vi "LEP_RV_MemoryMap_Default.vi"(8 "error in (no error)":errorcluster, 11 "VI Path":path) -> (0 "error out":errorcluster, 3 "VI Config":T1)   [LabVIEW 2011]
doc: "Define default memory mapping for the Axiom CMD565 target."
uses:
  <vilib>/LabVIEW Targets/Embedded/Utilities/MemMap/EMB_Utility_MemMap_VI_Config.ctl
  <vilib>/LabVIEW Targets/Embedded/Utilities/MemMap/EMB_Utility_MemMap_VI_Type.ctl
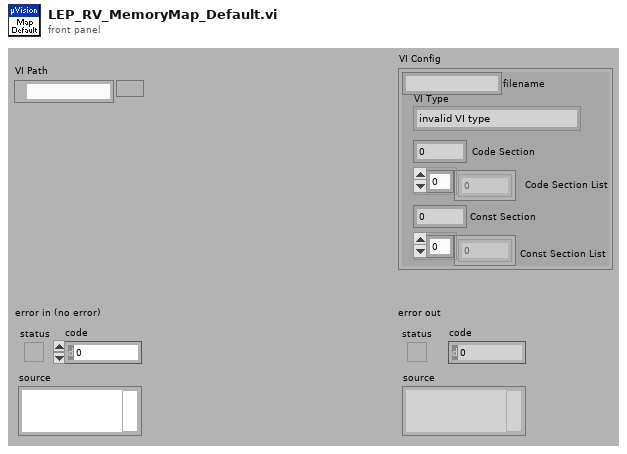
[diagram p1: front panel]
types:
  T1 = typedef "EMB_Utility_MemMap_VI_Config.ctl" = cluster{"filename":string, "Code Section":i32, "Code Section List":i32[], "Const Section":i32, "Const Section List":i32[], "VI Type":T2}
  T2 = typedef "EMB_Utility_MemMap_VI_Type.ctl" = enum32{"invalid VI type", "Standard VI", "Control VI", "Global VI", "Polymorphic VI", "Configuration VI", "SubSystem"}
  T3 = enum32{"invalid VI type", "Standard VI", "Control VI", "Global VI", "Polymorphic VI", "Configuration VI", "SubSystem", "Facade VI", "Method VI", "Statechart Diagram VI"}
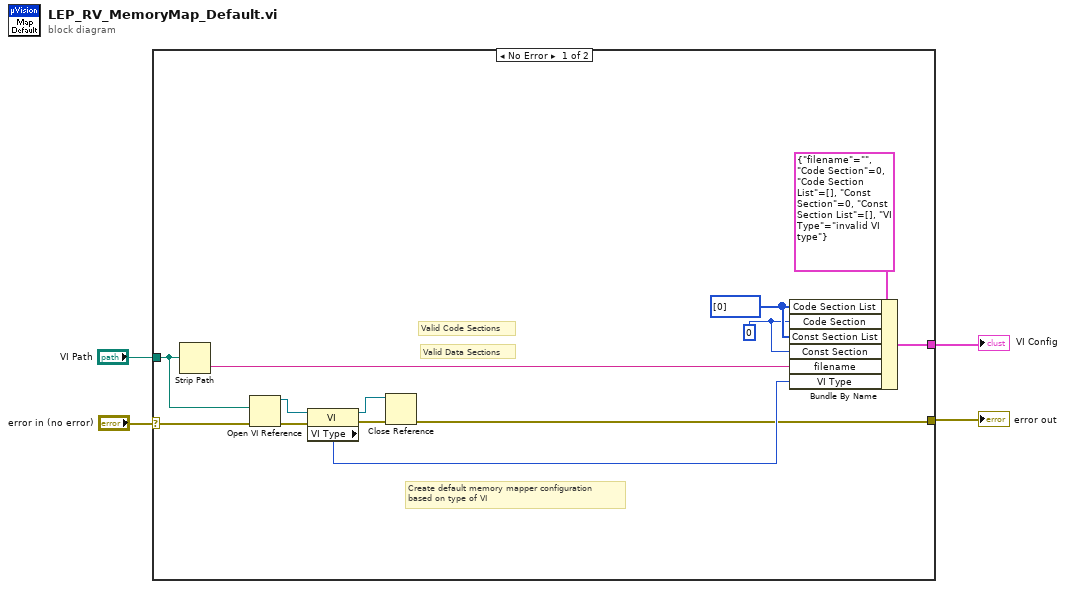
[diagram p0: block diagram]
diagram:
  n1 = case shown="No Error" "error in (no error)" {
    selector: "error in (no error)" -> [w16 w18]
    tunnel: [w7 w18] -> w3
    tunnel: "VI Path" -> [w8 _]
    tunnel: [w17 _] -> w1
    frame No Error {
      w6 = i32[] [0] ("Code Section List")
      w5 = 0 ("Code Section")
      # "Valid Data Sections"
      # "Valid Code Sections"
      # "Create default memory mapper configuration\nbased on type of VI"
      n2 = Strip Path(path=w8) -> (name=w13:string)  [unwired: 1 out]
      n3 = Open VI Reference(vi path=w8, error in (no error)=w16) -> (vi reference=w14:refnum<vi>, error out=w15:errorcluster)  [unwired: 4 in]
      n4 = property class="VI"(reference=w14, error in=w15) -> (reference out=w11:refnum<vi>, error out=w12:errorcluster, "VI Type"=w10:T3)
      n5 = Close Reference(reference=w11, error in (no error)=w12) -> (error out=w7:errorcluster)
      n6 = Bundle By Name(cluster=T1 {"filename"="", "Code Section"=0, "Code Section List"=[], "Const Section"=0, "Const Section List"=[], "VI Type"=enum."invalid VI type"} ("VI Config"), "Code Section List"=w6, "Code Section"=w5, "Const Section List"=w6, "Const Section"=w5, "filename"=w13, "VI Type"=w10) -> (w17:T1)
    }
    frame Error {
    }
  }
  "error out" <- w3
  "VI Config" <- w1
